vi "String to Connection.vi"(11 "String":string) -> (3 "Connection":T1)   [LabVIEW 2017, in "Switch Scripting.lvlib"]
uses:
  Switch Scripting.lvlib
  Shared/Connection.ctl
  <vilib>/regexp/Match Regular Expression.xnode
  Shared/Routing and Faulting Shared.lvlib
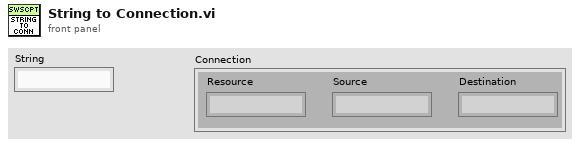
[diagram p1: front panel]
types:
  T1 = typedef "Routing and Faulting Shared.lvlib/Connection.ctl" = cluster{"Resource":string, "Source":string, "Destination":string}
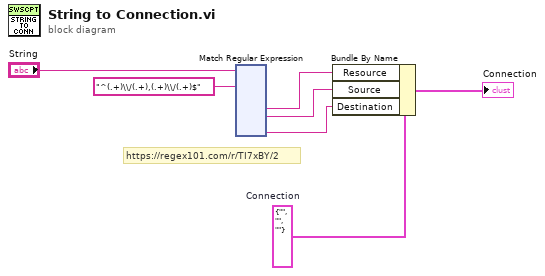
[diagram p0: block diagram]
diagram:
  w5 = T1 {"Resource"="", "Source"="", "Destination"=""}  # Connection
  # "https://regex101.com/r/TI7xBY/2"
  n1 = xnode "Match Regular Expression"("input string"="String", "regular expression"="^(.+)\\/(.+),(.+)\\/(.+)$" ("search string")) -> ("submatch 1"=w3:string, "submatch 2"=w2:string, "submatch 4"=w1:string)  [unwired: 4 in, 6 out]
  n2 = Bundle By Name(cluster=w5, "Resource"=w3, "Source"=w2, "Destination"=w1) -> (→"Connection":T1)
